vi "Set Build Specs.vi"(8 "error in":errorcluster, 11 "consumer data":T1) -> (0 "error out":errorcluster, 3 "consumer data out":T1)   [LabVIEW 2020, in "Template Tool.lvlib"]
uses:
  Template Tool.lvlib
  Consumer Data.ctl
  Project Build Specs.ctl
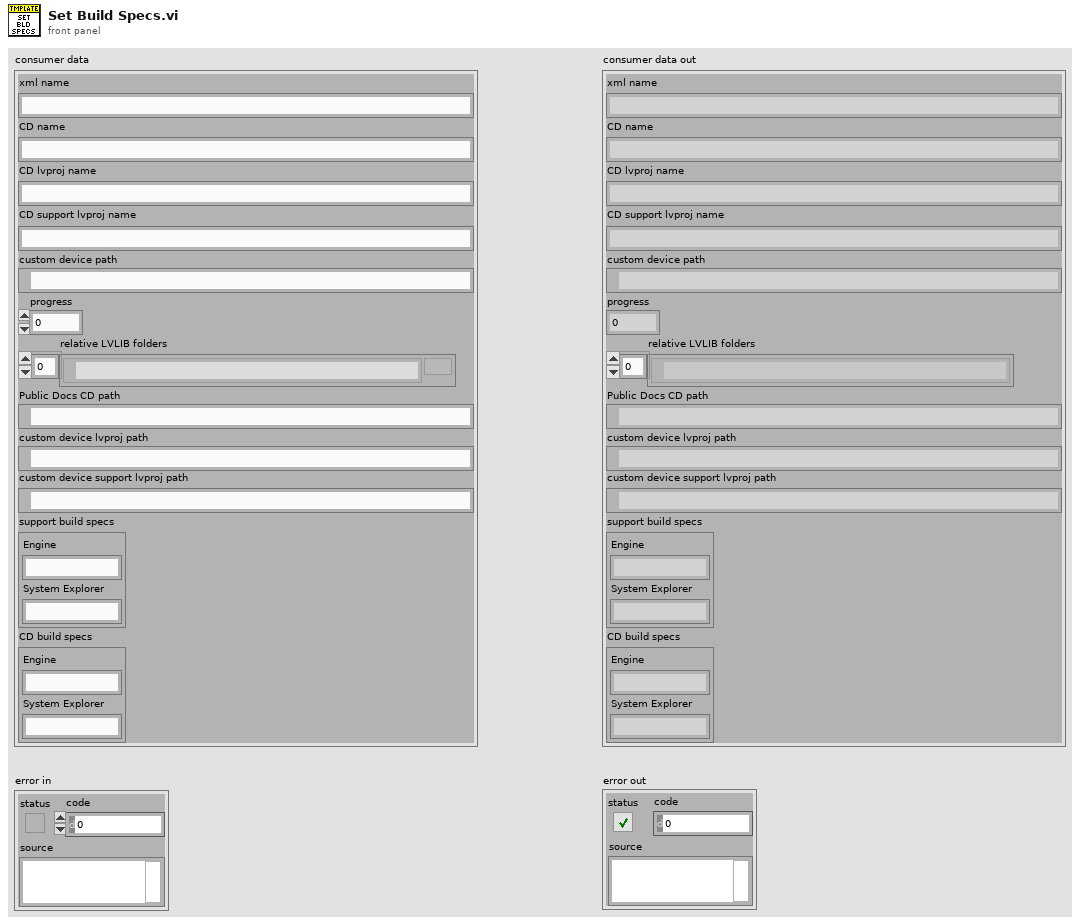
[diagram p1: front panel]
types:
  T1 = typedef "Template Tool.lvlib/Consumer Data.ctl" = cluster{"xml name":string, "CD name":string, "CD lvproj name":string, "CD support lvproj name":string, "custom device path":path, "progress":u8, "relative LVLIB folders":path[], "Public Docs CD path":path, "custom device lvproj path":path, "custom device support lvproj path":path, "support build specs":T2, "CD build specs":T2}
  T2 = typedef "Template Tool.lvlib/Project Build Specs.ctl" = cluster{"Engine":string, "System Explorer":string}
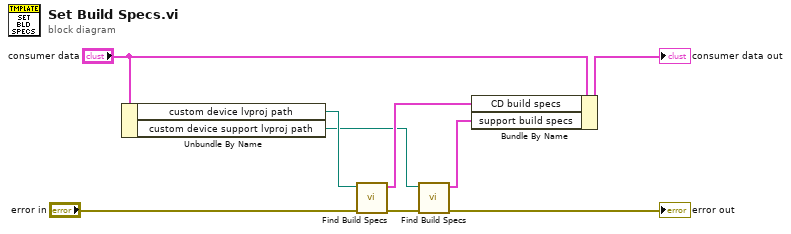
[diagram p0: block diagram]
diagram:
  n1 = Unbundle By Name("consumer data") -> ("custom device lvproj path"=w8:path, "custom device support lvproj path"=w3:path)
  n2 = call "Find Build Specs.vi"("error in"="error in", "project path"=w8) -> ("error out"=w4:errorcluster, "build specs"=w5:T2)  [unwired: 8 in]
  n3 = call "Find Build Specs.vi"("error in"=w4, "project path"=w3) -> ("error out"=→"error out":errorcluster, "build specs"=w2:T2)  [unwired: 8 in]
  n4 = Bundle By Name(cluster="consumer data", "CD build specs"=w5, "support build specs"=w2) -> (→"consumer data out":T1)
